vi "Launch as Nested.vi"(8 "error in (no error)":errorcluster, 9 "Log":string, 10 "Log Root":path, 11 "Parent in":refnum<class "Module.lvclass">) -> (0 "error out":errorcluster, 2 "MessageQ":refnum<class "MessageQ.lvclass">, 3 "Parent":refnum<class "Module.lvclass">)   [LabVIEW 2020, in "VolatusData.lvlib" / "Log Preparer Module.lvclass"]
uses:
  Log Preparer Module.lvclass
  Log Preparer Module.lvclass/Log Preparer Module.ctl
  Volatus/Module/Module.lvclass
  VolatusConfig/VolatusConfigElement/VolatusConfigElement.lvclass
  C:/dev/lv20CE/relink/lv-volatus/Volatus/Module/Module.lvclass
  C:/dev/lv20CE/relink/lv-volatus/VolatusData/Log Preparer Module/Log Preparer Module.lvclass
  Volatus/MessageQ/MessageQ.lvclass
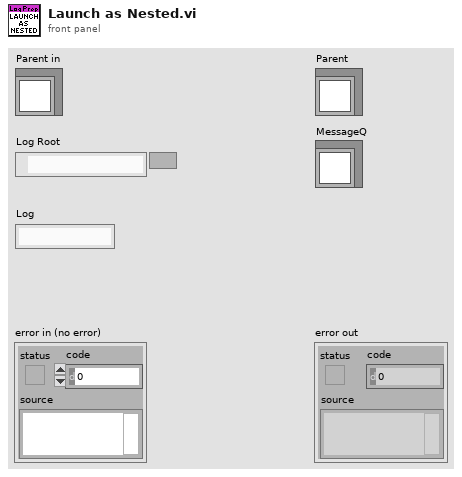
[diagram p1: front panel]
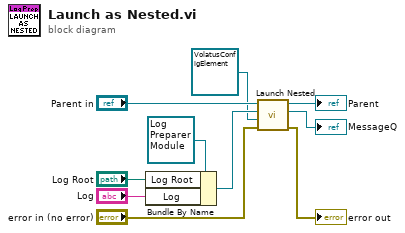
[diagram p0: block diagram]
diagram:
  n1 = Bundle By Name(cluster=refnum<class "Log Preparer Module.lvclass"> refnum ("Log Preparer Module in"), "Log Root"="Log Root", "Log"="Log") -> (w7:refnum<class "Log Preparer Module.lvclass">)
  n2 = call "Launch Nested.vi"("error in (no error)"="error in (no error)", "Config Element"=refnum<class "VolatusConfigElement.lvclass"> refnum, "Nested Module"=w7, "Parent in"="Parent in") -> ("error out"=→"error out":errorcluster, "MessageQ"=→"MessageQ":refnum<class "MessageQ.lvclass">, "Parent out"=→"Parent":refnum<class "Module.lvclass">)  [unwired: 5 in]
